vi "WiFi Setup.vi"(0 "IP address":u8[](array[numeric])=[127, 0, 0, 1], 1 "Gateway address":u8[](array[numeric])=[127, 0, 0, 3], 2 "Subnet mask":u8[](array[numeric])=[255, 255, 255, 0], 3 "DNS address":u8[](array[numeric])=[1, 2, 3, 4], 7 "WiFi Mode":T1(ring)=enum."WIFI_AP", 11 "Error In":errorcluster) -> (15 "Error Out":errorcluster)   [LabVIEW 2014, in "ESP8266 WiFi Wrapper.lvlib"]
doc: "Sets wifi network with given IP address, MAC adress, gateway and DNS. It is enough to let DNS 0.0.0.0"
uses:
  ESP8266 WiFi Wrapper.lvlib
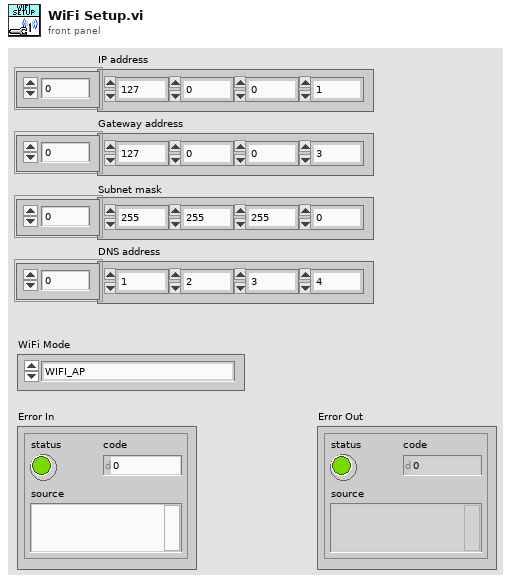
[diagram p1: front panel]
types:
  T1 = enum16{"WIFI_OFF", "WIFI_STA", "WIFI_AP", "WIFI_AP_STA"}
  T2 = enum8{"WIFI_OFF", "WIFI_STA", "WIFI_AP", "WIFI_AP_STA"}
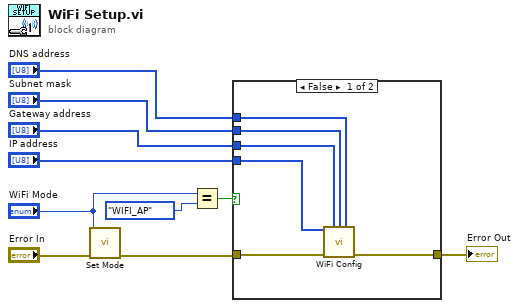
[diagram p0: block diagram]
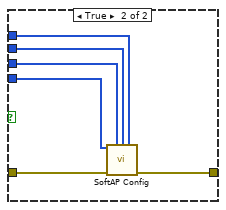
[diagram p2: hidden frame]
diagram:
  n1 = call "Set Mode.vi"("Error In"="Error In", "WiFi Server Mode"="WiFi Mode") -> ("Error Out"=w10:errorcluster)  [unwired: 9 in]
  n2 = Equal?(x="WiFi Mode", y=T2."WIFI_AP" ("Enum")) -> (x = y?=w6:bool)
  n3 = case shown="False" w6 {
    tunnel: w10 -> [w16 w22]
    tunnel: [w15 w21] -> w5
    tunnel: "IP address" -> [w14 w20]
    tunnel: "Gateway address" -> [w13 w19]
    tunnel: "Subnet mask" -> [w12 w18]
    tunnel: "DNS address" -> [w11 w17]
    frame False {
      n4 = call "WiFi Config.vi"("IP address"=w14, "Gateway address"=w13, "Subnet mask"=w12, "DNS address"=w11, "Error In"=w16) -> ("Error Out"=w15:errorcluster)  [unwired: 10 in]
    }
    frame True {
      n5 = call "SoftAP Config.vi"("IP address"=w20, "Gateway address"=w19, "Subnet mask"=w18, "DNS address"=w17, "Error In"=w22) -> ("Error Out"=w21:errorcluster)  [unwired: 10 in]
    }
  }
  "Error Out" <- w5
